vi "UpdateWeek.vi"() -> ()   [LabVIEW 2022 SP3]
uses:
  TypeDefs/Comic.ctl
  TypeDefs/Character.ctl
  TypeDefs/Creator.ctl
  TypeDefs/Variant.ctl
  14f7bc4a-da15-464d-b3b9-b5eb56e3d304.vi
  <vilib>/Comparison/Less/Less Functor/Less Functor.lvclass
panel:
  out "error out":errorcluster
  out "Current Comic":string
  out "Array":T1[](array[typedef]) {"Cover Price" format="$%.2g"}
  in  "error in":errorcluster
  in  "WeeklyFile":path
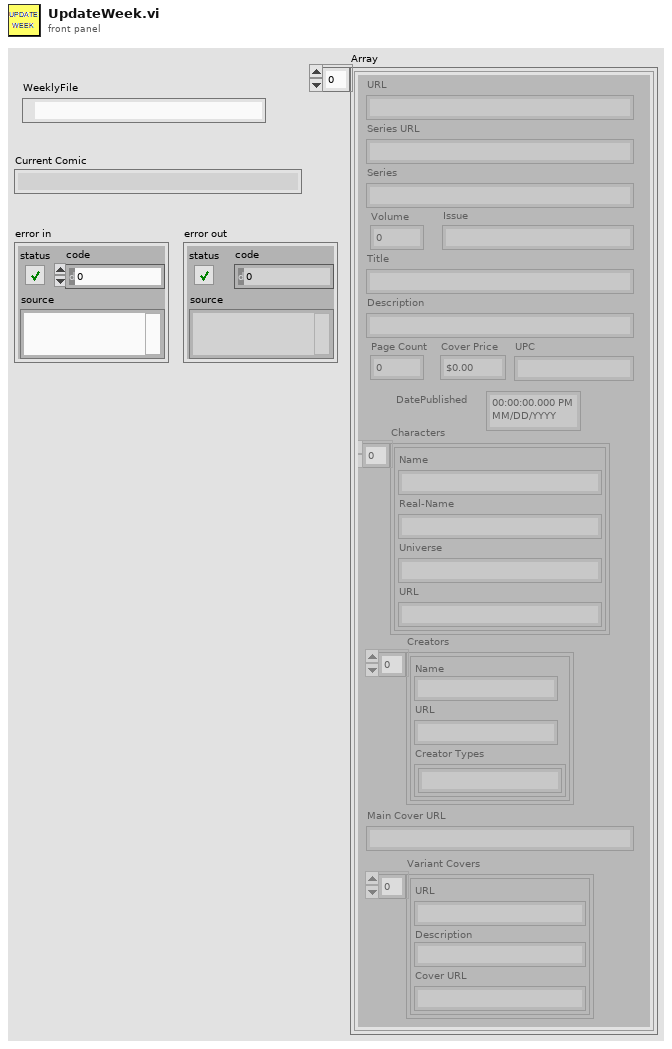
[diagram p1: front panel]
types:
  T1 = typedef "Comic.ctl" = cluster{"URL":string, "Series URL":string, "Series":string, "Volume":i32, "Issue":string, "Title":string, "Description":string, "Page Count":i32, "Cover Price":dbl, "UPC":string, "Characters":T2[], "Creators":T3[], "Main Cover URL":string, "Variant Covers":T4[], "DatePublished":timestamp}
  T2 = typedef "Character.ctl" = cluster{"Name":string, "Real-Name":string, "Universe":string, "URL":string}
  T3 = typedef "Creator.ctl" = cluster{"Name":string, "URL":string, "Creator Types":string[]}
  T4 = typedef "Variant.ctl" = cluster{"URL":string, "Description":string, "Cover URL":string}
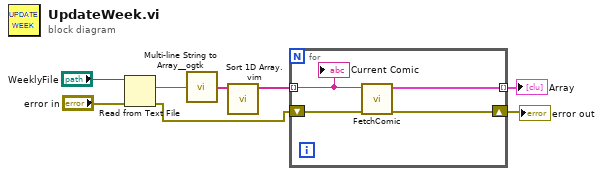
[diagram p0: block diagram]
diagram:
  n1 = Read from Text File(file (use dialog)="WeeklyFile", error in="error in") -> (text=w7:string, error out=w4:errorcluster)  [unwired: 2 in, 2 out]
  n2 = call <userlib>:"Multi-line String to Array__ogtk.vi"("string"=w7) -> ("lines"=w5:string[])
  n3 = call "Sort 1D Array.vim"("unsorted array"=w5) -> ("sorted array"=w2:string[])  [unwired: 10 in]
  n4 = for {
    tunnel: w2 -> [w12] mode=indexing
    shift-right: [w10] -> w1
    shift-left: w4 -> [w11]
    tunnel: [w9] -> w3 mode=indexing
    n5 = call "FetchComic.vi"("error in (no error)"=w11, "ComicURL"=w12) -> ("error out"=w10:errorcluster, "Comic"=w9:T1)  [unwired: 8 in]
    "Current Comic" <- w12
  }
  "Array" <- w3
  "error out" <- w1
